vi "Repeat Until Timeout.vi"(7 "Name":string="Repeat Until Timeout", 8 "On Timeout Status":T1, 9 "Timeout (s)":dbl, 10 "Finish On":T2, 11 "Node In":refnum<class "abs_Node.lvclass">) -> (3 "Node Out":refnum<class "abs_Node.lvclass">)   [LabVIEW 2021, in "BT.lvlib"]
uses:
  BT.lvlib
  Support/Nodes/Decorators/Repeat Until Timeout/Repeat Until Timeout.lvclass
  C:/Users/Tim/Documents/GitHub/LV_Behaviour_Tree/Source/Support/abs_Node/abs_Node.lvclass
  Support/Nodes/abs_Node/abs_Node.lvclass
  Support/Nodes/Decorators/Repeater/Support/Finish On - Type.ctl
  Support/Nodes/Decorators/Repeater/Repeater.lvclass
  Support/Nodes/Decorators/Repeat Until Timeout/Support/On Timeout Status - Type.ctl
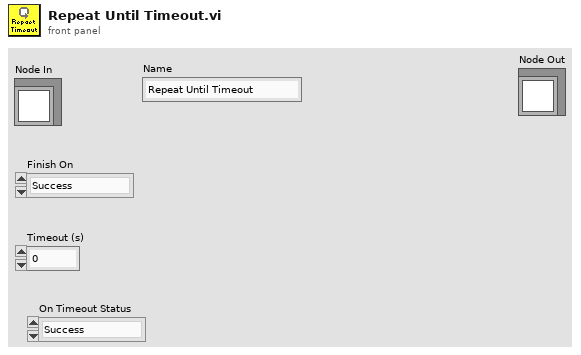
[diagram p1: front panel]
types:
  T1 = typedef "BT.lvlib/Repeat Until Timeout.lvclass/On Timeout Status - Type.ctl" = enum16{"Success", "Failure"}
  T2 = typedef "BT.lvlib/Repeater.lvclass/Finish On - Type.ctl" = enum16{"Success", "Failure", "Never"}
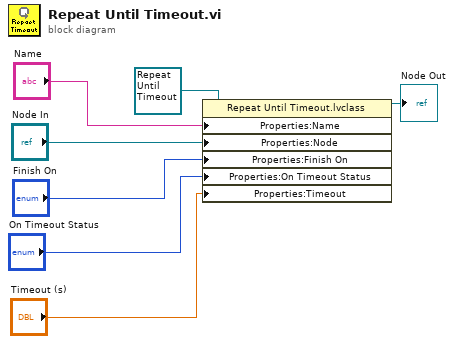
[diagram p0: block diagram]
diagram:
  n1 = property class="Repeat Until Timeout.lvclass"(reference=refnum<class "Repeat Until Timeout.lvclass"> refnum ("BT.lvlib:Repeat Until Timeout.lvclass"), "Properties:Name"="Name", "Properties:Node"="Node In", "Properties:Finish On"="Finish On", "Properties:On Timeout Status"="On Timeout Status", "Properties:Timeout"="Timeout (s)") -> (reference out=→"Node Out":refnum<class "Repeat Until Timeout.lvclass">)  [unwired: 1 in, 1 out]
